vi "Keithley2612b_IV_NOT.vi"(0 "VISA resource name":refnum<visa-resource-name>, 1 "Channel (Channel A) 2":T1, 3 "XY Graph Ref In":refnum<vi>, 4 "Channel (Channel A)":T1, 5 "error in (no error)":errorcluster, 6 "Source Function (Current)":enum32{"Current", "Voltage"}(ring)=enum."Voltage", 7 "Source Function (Current) 2":enum32{"Current", "Voltage"}(ring)=enum."Voltage", 8 "Appand to Exist File":bool, 10 "Write to Text File?":bool, 11 "Reverse Sweep":bool, 12 "Delay (s) 2":dbl, 13 "Current Limit 2":dbl=1.0, 14 "Error Query (False)":bool, 15 "Start Voltage 2":dbl, 17 "End Voltage 2":dbl, 18 "Step Size 2":dbl) -> (19 "error out":errorcluster)   [LabVIEW 2016]
doc: "This example shows how to configure the source and take a measurement."
uses:
  <instrlib>/Keithley 2600 Series/Public/Channel.ctl
  <vilib>/express/express shared/transition.llb/Dynamic To Waveform Array.vi
  <vilib>/express/express signal manip/GetorSetDDTAttributes/Set DDT Attributes/SetT0.vi
  <vilib>/express/express shared/transition.llb/Waveform Array To Dynamic.vi
  <vilib>/express/express signal manip/GetorSetDDTAttributes/Set DDT Attributes/Set DDT Properties.xnode
  <instrlib>/Keithley 2600 Series/Keithley 2600 Series.lvlib
panel:
  out "XY Graph":cluster{"Y":dbl[], "Y":dbl[]}[](graph)
  out "Current Output 2":string
  out "Voltage Output 2":string
  out "Current Number Past 2":dbl
  out "Current Number Past":dbl
  out "Voltage Output":string
  out "Current Output":string
  # "Gate Voltage"
  # "Drain Voltage"
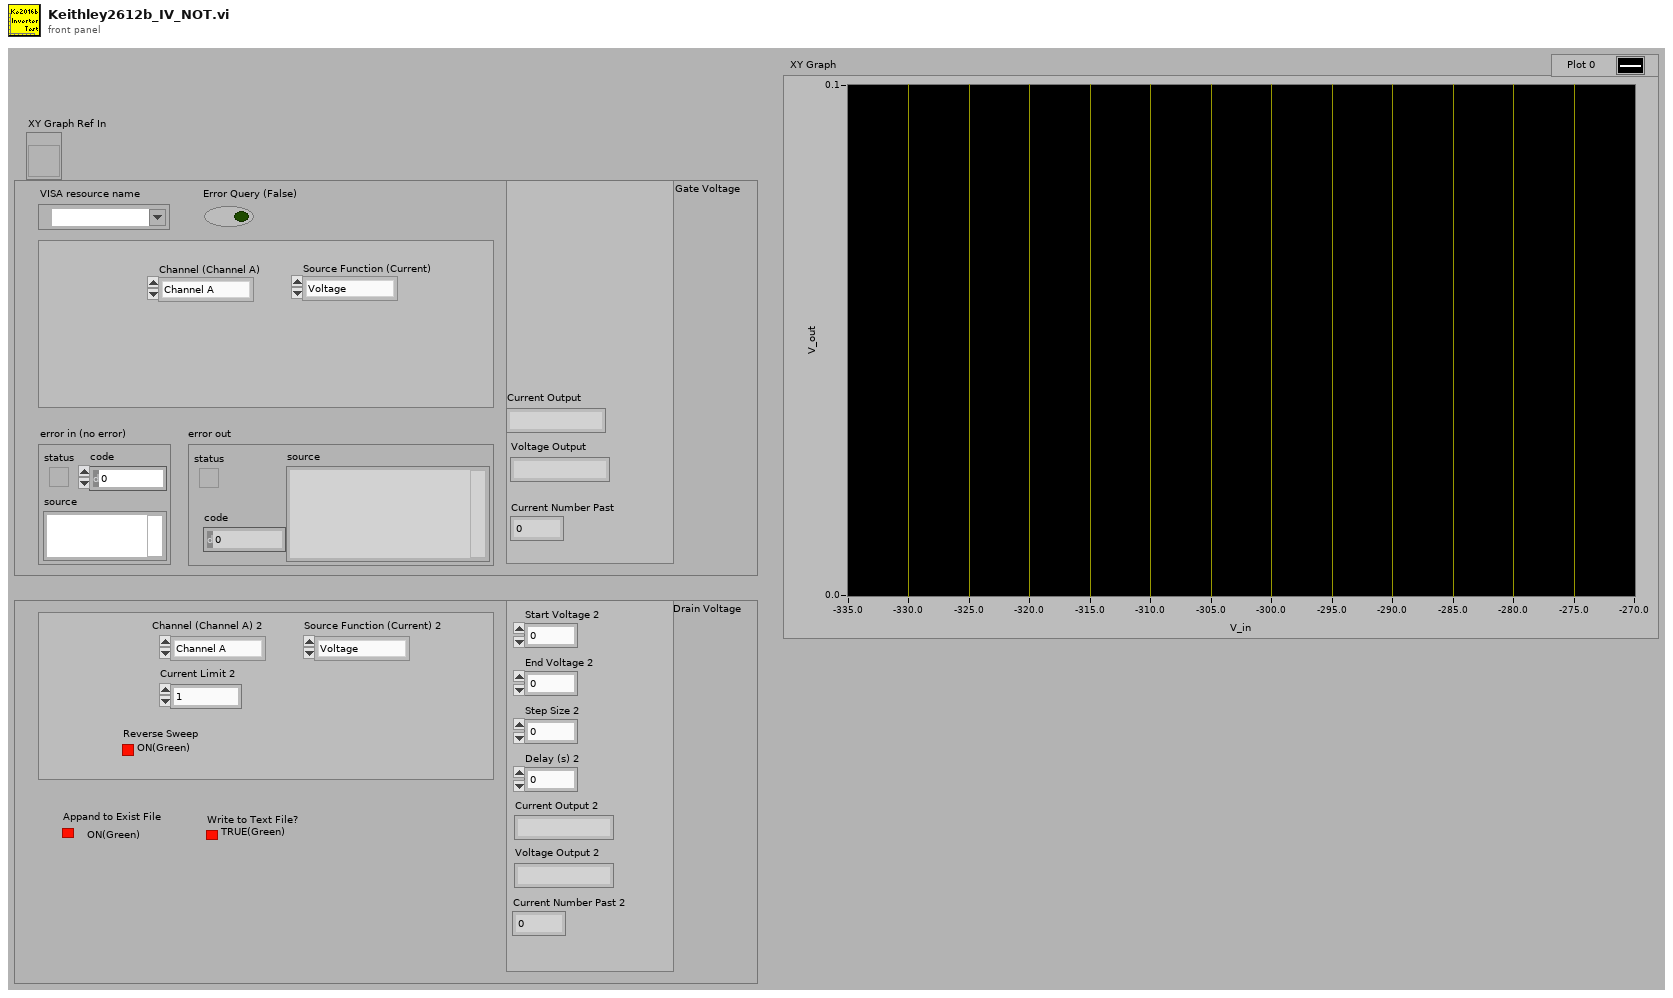
[diagram p1: front panel]
types:
  T1 = typedef "Keithley 2600 Series.lvlib/Channel.ctl" = enum32{"Channel A", "Channel B"}
  T2 = typedef "NI_Matrix.lvlib/RealMatrix.ctl" = dbl[][]
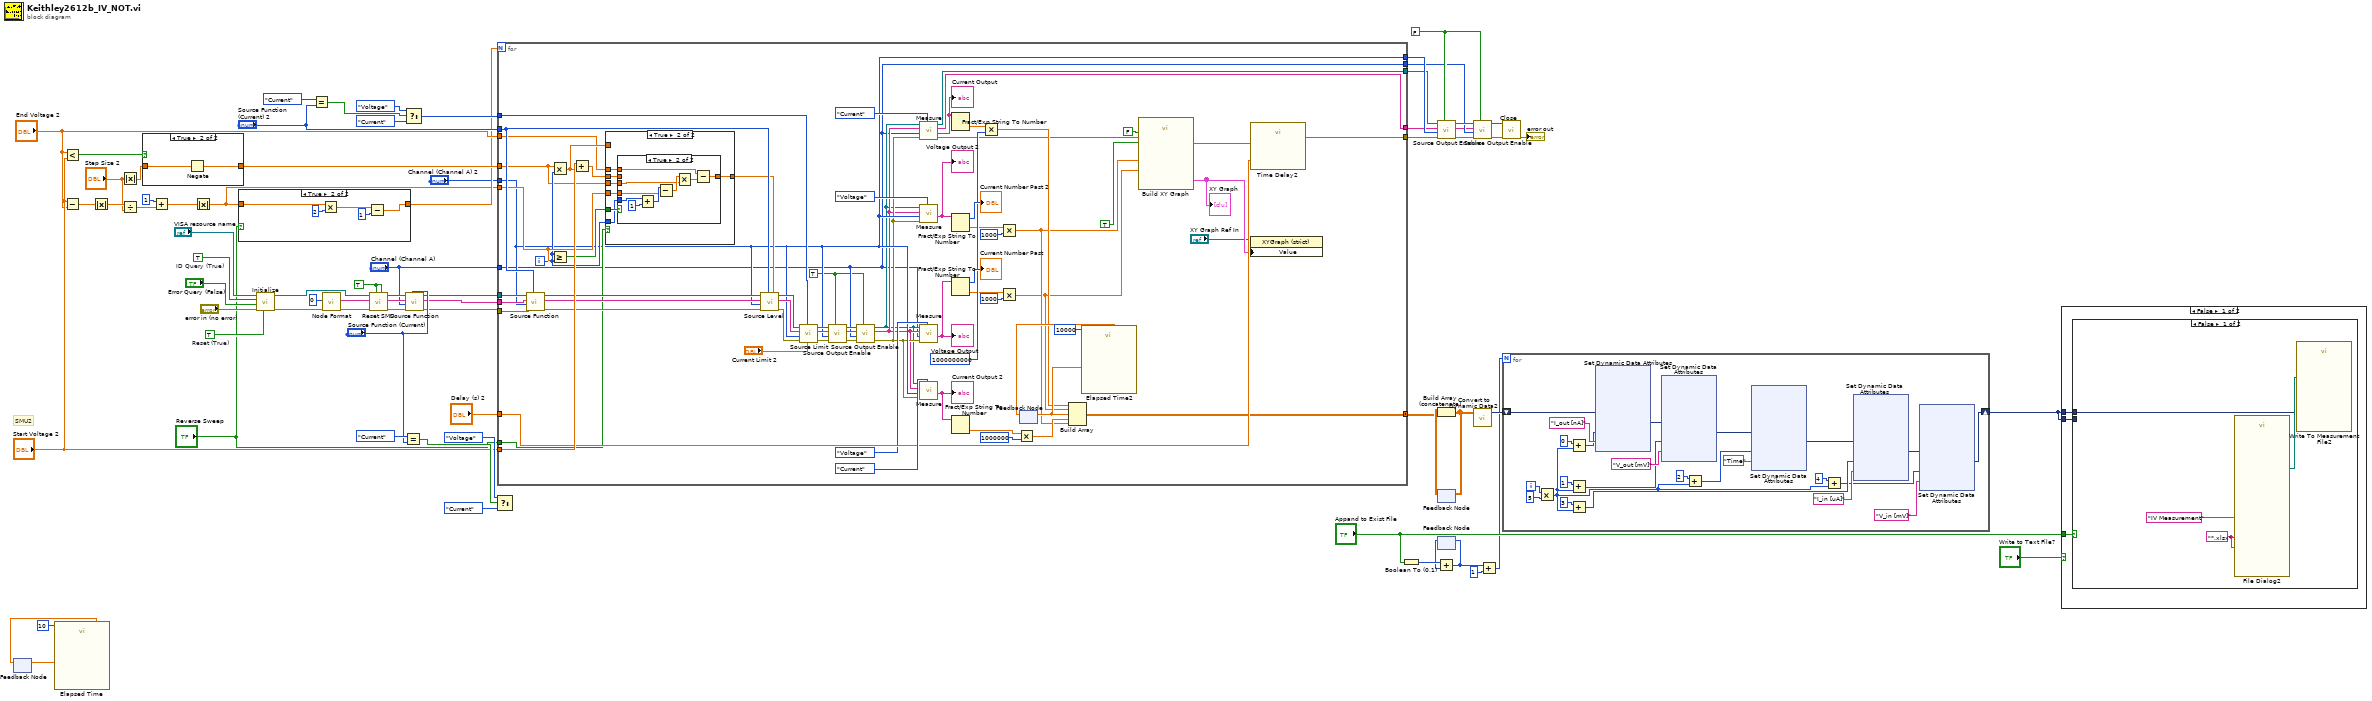
[diagram p0: block diagram]
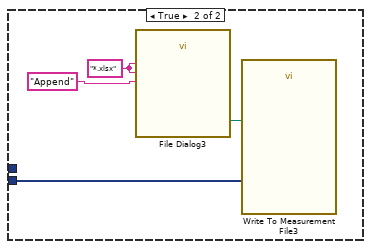
[diagram p2: hidden frame]
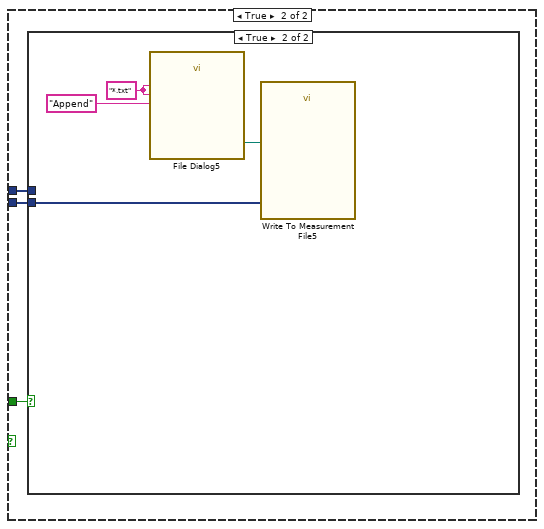
[diagram p3: hidden frame]
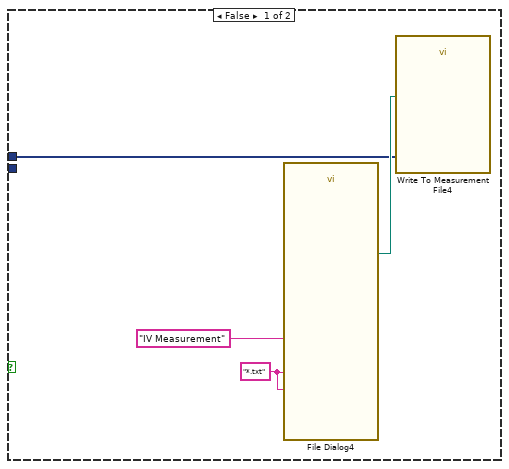
[diagram p4: hidden frame]
diagram:
  w51 = TRUE
  w38 = FALSE ("Output (Off)")
  w69 = TRUE  # Reset (True)
  w72 = TRUE  # ID Query (True)
  # "SMU2"
  n1 = feedback #1() -> (w25:dbl)  [unwired: 1 in]
  n2 = call "Elapsed Time"("Time Target (s)"=10, "Set Start Time (s)"=w25) -> ("Elapsed Time (s)"=w27:dbl)  [unwired: 10 in, 7 out]
  n3 = feedback-in #1(w27) -> ()
  n4 = Less?(x="End Voltage 2", y="Start Voltage 2") -> (x < y?=w36:bool)
  n5 = Subtract(x="Start Voltage 2", y="End Voltage 2") -> (x-y=w47:dbl)
  n6 = Absolute Value(x=w47) -> (abs(x)=w46:dbl)
  n7 = Absolute Value(x="Step Size 2") -> (abs(x)=w34:dbl)
  n8 = Divide(x=w46, y="Step Size 2") -> (x/y=w44:dbl)
  n9 = case shown="True" w36 {
    tunnel: w34 -> [w73 w74]
    tunnel: [w73 w75] -> w35
    frame False {
    }
    frame True {
      n10 = Negate(x=w74) -> (-x=w75:dbl)
    }
  }
  n11 = Add(x=1, y=w44) -> (x+y=w32:dbl)
  n12 = Absolute Value(x=w32) -> (abs(x)=w29:dbl)
  n13 = case shown="True" "Reverse Sweep" {
    tunnel: w29 -> [w76 w81]
    tunnel: [w76 w79] -> w30
    frame False {
    }
    frame True {
      n14 = Multiply(x=w81, y=2) -> (x*y=w78:dbl)
      n15 = Subtract(x=w78, y=1) -> (x-y=w79:dbl)
    }
  }
  n16 = call <instrlib>:"Initialize.vi"("Reset (True)"=w69, "error in (no error)"="error in (no error)", "Error Query (False)"="Error Query (False)", "ID Query (True)"=w72, "VISA resource name"="VISA resource name") -> ("error out"=w59:errorcluster, "VISA resource name out"=w52:refnum<visa-resource-name>)  [unwired: 1 in, 4 out]
  n17 = Equal?(x=enum32{"Current", "Voltage"}."Current", y="Source Function (Current) 2") -> (x = y?=w57:bool)
  n18 = call <instrlib>:"Node Format.vi"("error in"=w59, "Node (0-64)"=i8 0) -> ("error out"=w65:errorcluster, "Formatted Node"=w66:string)  [unwired: 8 out]
  n19 = call <instrlib>:"Reset SMU.vi"("SMU B (No)"=w51, "SMU A (No)"=w51, "error in (no error)"=w65, "Node In"=w66, "VISA resource name"=w52) -> ("error out"=w50:errorcluster, "Node Out"=w48:string, "VISA resource name out"=w49:refnum<visa-resource-name>)  [unwired: 4 out]
  n20 = Equal?(x=enum32{"Current", "Voltage"}."Current", y="Source Function (Current)") -> (x = y?=w67:bool)
  n21 = Select(t=enum32{"Current", "Voltage"}."Voltage" ("x"), s=w57, f=enum32{"Current", "Voltage"}."Current") -> (s? t:f=w41:enum32{"Current", "Voltage"})
  n22 = call <instrlib>:"Source Function.vi"("Function (Current)"="Source Function (Current)", "error in (no error)"=w50, "Channel (Channel A)"="Channel (Channel A)", "Node In"=w48, "VISA resource name"=w49) -> ("error out"=w1:errorcluster, "Node Out"=w2:string, "VISA resource name out"=w3:refnum<visa-resource-name>)  [unwired: 4 out]
  n23 = Select(t=enum32{"Current", "Voltage"}."Voltage" ("x"), s=w67, f=enum32{"Current", "Voltage"}."Current") -> ()  [unwired: 1 out]
  n24 = for {
    N: w30 -> [_]
    tunnel: w35 -> [w121]
    tunnel: "Start Voltage 2" -> [w144]
    tunnel: w41 -> [w143]
    tunnel: [w142] -> w15
    tunnel: w3 -> [w133]
    tunnel: "Delay (s) 2" -> [w135]
    tunnel: "Source Function (Current) 2" -> [w130]
    tunnel: [w129] -> w23 mode=concatenating
    tunnel: "End Voltage 2" -> [w120]
    tunnel: "Reverse Sweep" -> [w128]
    tunnel: w29 -> [w124]
    tunnel: w2 -> [w102]
    tunnel: "Channel (Channel A) 2" -> [w101]
    tunnel: "Channel (Channel A)" -> [w92]
    tunnel: [w101] -> w20
    tunnel: [w92] -> w19
    tunnel: [w100] -> w17
    tunnel: [w99] -> w16
    tunnel: w1 -> [w82]
    i -> [w122]
    w91 = TRUE ("Output (Off)")
    n25 = call <instrlib>:"Source Function.vi"("Function (Current)"=w130, "error in (no error)"=w82, "Channel (Channel A)"=w101, "Node In"=w102, "VISA resource name"=w133) -> ("error out"=w134:errorcluster, "Node Out"=w132:string, "VISA resource name out"=w131:refnum<visa-resource-name>)  [unwired: 4 out]
    n26 = Multiply(x=w121, y=w122) -> (x*y=w123:dbl)
    n27 = Greater Or Equal?(x=w122, y=w124) -> (x >= y?=w125:bool)
    n28 = Add(x=w144, y=w123) -> (x+y=w127:dbl)
    n29 = case shown="True" w128 {
      tunnel: w125 -> [_ w159]
      tunnel: w127 -> [w152 w158]
      tunnel: [w152 w157] -> w126
      tunnel: w124 -> [_ w156]
      tunnel: w123 -> [_ _]
      tunnel: w122 -> [_ w155]
      tunnel: w121 -> [_ w154]
      tunnel: w120 -> [_ w153]
      frame False {
      }
      frame True {
        n30 = case shown="True" w159 {
          tunnel: w158 -> [w160 _]
          tunnel: [w160 w161] -> w157
          tunnel: w156 -> [_ w168]
          tunnel: w155 -> [_ w167]
          tunnel: w154 -> [_ w164]
          tunnel: w153 -> [_ w162]
          frame False {
          }
          frame True {
            n31 = Add(x=w167, y=1) -> (x+y=w169:i32)
            n32 = Subtract(x=w169, y=w168) -> (x-y=w165:dbl)
            n33 = Multiply(x=w165, y=w164) -> (x*y=w163:dbl)
            n34 = Subtract(x=w162, y=w163) -> (x-y=w161:dbl)
          }
        }
      }
    }
    n35 = call <instrlib>:"Source Level.vi"("Level (0.000)"=w126, "Function (Current)"=w130, "error in (no error)"=w134, "Channel (Channel A)"=w101, "Node In"=w132, "VISA resource name"=w131) -> ("error out"=w145:errorcluster, "Node Out"=w149:string, "VISA resource name out"=w146:refnum<visa-resource-name>)  [unwired: 3 out]
    n36 = call <instrlib>:"Source Limit.vi"("Limit (0.000)"="Current Limit 2", "Function (Current)"=w143, "error in (no error)"=w145, "Channel (Channel A)"=w101, "Node In"=w149, "VISA resource name"=w146) -> ("error out"=w148:errorcluster, "Node Out"=w150:string, "VISA resource name out"=w147:refnum<visa-resource-name>)  [unwired: 3 out]
    n37 = call <instrlib>:"Source Output Enable.vi"("Output (Off)"=w91, "error in (no error)"=w148, "Channel (Channel A)"=w101, "Node In"=w150, "VISA resource name"=w147) -> ("error out"=w97:errorcluster, "Node Out"=w95:string, "VISA resource name out"=w94:refnum<visa-resource-name>)  [unwired: 4 out]
    n38 = call <instrlib>:"Source Output Enable.vi"("Output (Off)"=w91, "error in (no error)"=w97, "Channel (Channel A)"=w92, "Node In"=w95, "VISA resource name"=w94) -> ("error out"=w98:errorcluster, "Node Out"=w96:string, "VISA resource name out"=w93:refnum<visa-resource-name>)  [unwired: 4 out]
    n39 = call <instrlib>:"Measure.vi"("Function (Current)"=enum32{"Current", "Voltage"}."Current" ("x"), "error in (no error)"=w98, "Channel (Channel A)"=w92, "Node In"=w96, "VISA resource name"=w93) -> ("error out"=w87:errorcluster, "Output"=w117:string, "Node Out"=w99:string, "VISA resource name out"=w100:refnum<visa-resource-name>)  [unwired: 2 in, 1 out]
    "Current Output" <- w117
    n40 = call <instrlib>:"Measure.vi"("Function (Current)"=enum32{"Current", "Voltage"}."Voltage" ("x"), "error in (no error)"=w98, "Channel (Channel A)"=w101, "Node In"=w96, "VISA resource name"=w93) -> ("Output"=w113:string)  [unwired: 2 in, 4 out]
    "Voltage Output 2" <- w113
    n41 = call <instrlib>:"Measure.vi"("Function (Current)"=enum32{"Current", "Voltage"}."Voltage" ("x"), "error in (no error)"=w98, "Channel (Channel A)"=w92, "Node In"=w96, "VISA resource name"=w93) -> ("Output"=w116:string)  [unwired: 2 in, 4 out]
    "Voltage Output" <- w116
    n42 = call <instrlib>:"Measure.vi"("Function (Current)"=enum32{"Current", "Voltage"}."Current" ("x"), "error in (no error)"=w98, "Channel (Channel A)"=w101, "Node In"=w96, "VISA resource name"=w93) -> ("Output"=w114:string)  [unwired: 2 in, 4 out]
    "Current Output 2" <- w114
    n43 = Fract/Exp String To Number(string=w117) -> (number=w107:dbl)  [unwired: 3 in, 1 out]
    n44 = Fract/Exp String To Number(string=w113) -> (offset past number=→"Current Number Past 2":i32, number=w103:dbl)  [unwired: 3 in]
    n45 = Fract/Exp String To Number(string=w116) -> (offset past number=→"Current Number Past":i32, number=w105:dbl)  [unwired: 3 in]
    n46 = Fract/Exp String To Number(string=w114) -> (number=w109:dbl)  [unwired: 3 in, 1 out]
    n47 = Multiply(x=w107, y=1000000000) -> (x*y=w111:dbl)
    n48 = Multiply(x=w103, y=1000) -> (x*y=w90:dbl)
    n49 = Multiply(x=w105, y=1000) -> (x*y=w89:dbl)
    n50 = Multiply(x=w109, y=1000000) -> (x*y=w108:dbl)
    n51 = feedback #2() -> (w136:dbl)  [unwired: 1 in]
    n52 = Build Array(w111, w89, w136, w108, w90) -> (w129:T2)
    n53 = call "Elapsed Time2"("Time Target (s)"=10000, "Set Start Time (s)"=w136) -> ("Elapsed Time (s)"=w139:dbl)  [unwired: 10 in, 7 out]
    n54 = feedback-in #2(w139) -> ()
    n55 = call "Build XY Graph"("Enable"=TRUE, "error in (no error)"=w87, "Reset"=FALSE, "Y Input"=w89, "X Input"=w90) -> ("error out"=w88:errorcluster, "XY Graph"=w84:cluster{"X":dbl[], "Y":dbl[]}[])  [unwired: 5 in]
    "XY Graph" <- w84
    n56 = call "Time Delay2"("error in (no error)"=w88, "Delay Time (s)"=w135) -> ("error out"=w142:errorcluster)  [unwired: 9 in]
    n57 = property class="XYGraph (strict)"(reference="XY Graph Ref In", "Value"=w84) -> ()  [unwired: 1 in, 2 out]
  }
  n58 = Boolean To (0,1)(Boolean="Appand to Exist File") -> (0, 1=w14:i16)
  n59 = call <instrlib>:"Source Output Enable.vi"("Output (Off)"=w38, "error in (no error)"=w15, "Channel (Channel A)"=w20, "Node In"=w16, "VISA resource name"=w17) -> ("error out"=w39:errorcluster, "Node Out"=w18:string, "VISA resource name out"=w40:refnum<visa-resource-name>)  [unwired: 4 out]
  n60 = feedback #3() -> (w24:T2)  [unwired: 1 in]
  n61 = Build Array (concatenate)(w24, w23) -> (w22:T2)
  n62 = feedback-in #3(w22) -> ()
  n63 = feedback #4() -> (w13:i16)  [unwired: 1 in]
  n64 = Add(x=w14, y=w13) -> (x+y=w11:i16)
  n65 = feedback-in #4(w11) -> ()
  n66 = call <instrlib>:"Source Output Enable.vi"("Output (Off)"=w38, "error in (no error)"=w39, "Channel (Channel A)"=w19, "Node In"=w18, "VISA resource name"=w40) -> ("error out"=w61:errorcluster, "VISA resource name out"=w62:refnum<visa-resource-name>)  [unwired: 5 out]
  n67 = call "Convert to Dynamic Data2"("2D Array"=w22) -> ("Dynamic Data Type"=w9:dynamicdata)  [unwired: 3 in]
  n68 = Add(x=w11, y=1) -> (x+y=w7:i32)
  n69 = call <instrlib>:"Close.vi"("error in (no error)"=w61, "VISA resource name"=w62) -> ("error out"=→"error out":errorcluster)  [unwired: 9 out]
  n70 = for {
    N: w7 -> [_]
    shift-right: [w183] -> w6
    shift-left: w9 -> [w184]
    i -> [w170]
    n71 = Multiply(x=w170, y=5) -> (x*y=w172:i32)
    n72 = Add(x=0, y=w172) -> (x+y=w180:i32)
    n73 = Add(x=1, y=w172) -> (x+y=w177:i32)
    n74 = Add(x=3, y=w172) -> (x+y=w174:i32)
    n75 = xnode "Set Dynamic Data Attributes"("Signals In"=w184, "Signal Index"=w180, "Signal Name"="I_out [nA]") -> ("Signals Out"=w185:dynamicdata)  [unwired: 1 in, 1 out]
    n76 = xnode "Set Dynamic Data Attributes"("Signals In"=w185, "Signal Index"=w177, "Signal Name"="V_out [mV]") -> ("Signals Out"=w186:dynamicdata)  [unwired: 1 in, 1 out]
    n77 = Add(x=2, y=w172) -> (x+y=w176:i32)
    n78 = xnode "Set Dynamic Data Attributes"("Signals In"=w186, "Signal Index"=w176, "Signal Name"="Time") -> ("Signals Out"=w187:dynamicdata)  [unwired: 1 in, 1 out]
    n79 = Add(x=4, y=w172) -> (x+y=w171:i32)
    n80 = xnode "Set Dynamic Data Attributes"("Signals In"=w187, "Signal Index"=w174, "Signal Name"="I_in [uA]") -> ("Signals Out"=w188:dynamicdata)  [unwired: 1 in, 1 out]
    n81 = xnode "Set Dynamic Data Attributes"("Signals In"=w188, "Signal Index"=w171, "Signal Name"="V_in [mV]") -> ("Signals Out"=w183:dynamicdata)  [unwired: 1 in, 1 out]
  }
  n82 = case shown="False" "Write to Text File?" {
    tunnel: "Appand to Exist File" -> [w260 w272]
    tunnel: w6 -> [w261 w271]
    tunnel: w6 -> [w259 w270]
    frame False {
      n83 = case shown="False" w260 {
        tunnel: w259 -> [w262 _]
        tunnel: w261 -> [_ w266]
        frame False {
          w265 = "*.xlsx"
          n84 = call "File Dialog2"("default name"="IV Measurement", "pattern (all files)"=w265, "pattern label"=w265) -> ("selected path"=w263:path)  [unwired: 9 in, 3 out]
          n85 = call "Write To Measurement File2"("Signals"=w262, "Filename"=w263) -> ()  [unwired: 15 in, 3 out]
        }
        frame True {
          w269 = "*.xlsx"
          n86 = call "File Dialog3"("button label"="Append", "pattern (all files)"=w269, "pattern label"=w269) -> ("selected path"=w268:path)  [unwired: 9 in, 3 out]
          n87 = call "Write To Measurement File3"("Signals"=w266, "Filename"=w268) -> ()  [unwired: 15 in, 3 out]
        }
      }
    }
    frame True {
      n88 = case shown="True" w272 {
        tunnel: w270 -> [w273 _]
        tunnel: w271 -> [_ w278]
        frame False {
          w276 = "*.txt"
          n89 = call "File Dialog4"("default name"="IV Measurement", "pattern (all files)"=w276, "pattern label"=w276) -> ("selected path"=w274:path)  [unwired: 9 in, 3 out]
          n90 = call "Write To Measurement File4"("Signals"=w273, "Filename"=w274) -> ()  [unwired: 15 in, 3 out]
        }
        frame True {
          w280 = "*.txt"
          n91 = call "File Dialog5"("button label"="Append", "pattern (all files)"=w280, "pattern label"=w280) -> ("selected path"=w279:path)  [unwired: 9 in, 3 out]
          n92 = call "Write To Measurement File5"("Signals"=w278, "Filename"=w279) -> ()  [unwired: 15 in, 3 out]
        }
      }
    }
  }
